vi "RotateView.vi"(8 "error in (no error)":errorcluster, 9 "Pitch":sgl, 10 "Yaw":sgl, 11 "3D Scene in":refnum<class "3D Scene.lvclass">) -> (0 "error out":errorcluster, 3 "3D Scene out":refnum<class "3D Scene.lvclass">)   [LabVIEW 2015, in "3D Scene.lvclass"]
uses:
  3D Scene.lvclass
  3D Scene.lvclass/3D Scene.ctl
  <vilib>/Analysis/baseanly.llb/Real A x B.vi
  <vilib>/Analysis/baseanly.llb/Vector x A.vi
  <vilib>/Analysis/NI_AALBase.lvlib
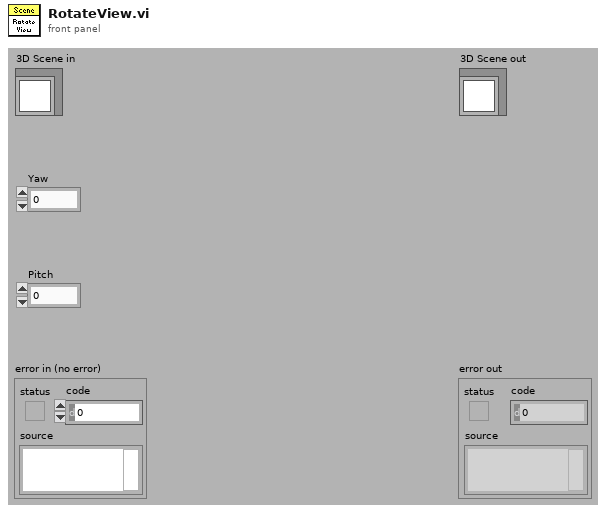
[diagram p1: front panel]
types:
  T1 = typedef "NI_Matrix.lvlib/RealMatrix.ctl" = dbl[][]
  T2 = typedef "3D Point.ctl" = cluster{"X":sgl, "Y":sgl, "Z":sgl}
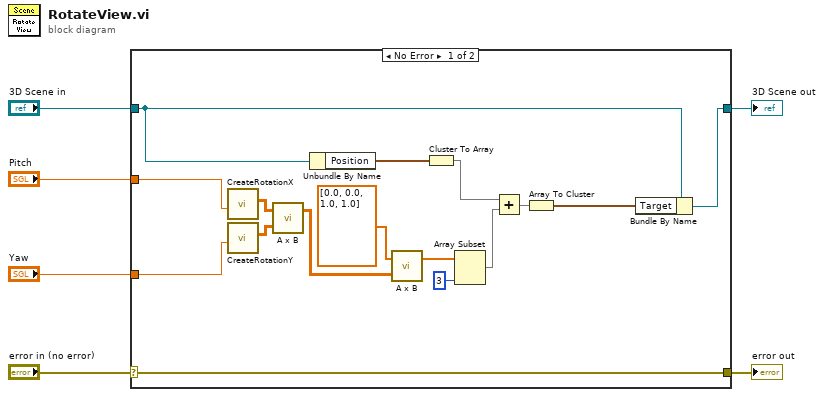
[diagram p0: block diagram]
diagram:
  n1 = case shown="No Error" "error in (no error)" {
    selector: "error in (no error)" -> [w22 w24]
    tunnel: [w22 w24] -> w5
    tunnel: [w16 w23] -> w3
    tunnel: "3D Scene in" -> [w17 w23]
    tunnel: "Pitch" -> [w19 _]
    tunnel: "Yaw" -> [w18 _]
    frame No Error {
      n2 = call "CreateRotationX.vi"("radians"=w19) -> ("modelview rotated"=w10:T1)  [unwired: 8 in, 2 out]
      n3 = call "CreateRotationY.vi"("radians"=w18) -> ("modelview rotated"=w9:T1)  [unwired: 8 in, 2 out]
      n4 = call-poly <vilib>:"A x B.vi"("B"=w9, "A"=w10) -> ("A x B"=w7:T1)  [unwired: 1 out]
      n5 = Unbundle By Name(w17) -> ("Position"=w20:T2)
      n6 = call-poly <vilib>:"A x B.vi"("Matrix A"=w7, "Vector V'"=dbl[] [0.0, 0.0, 1.0, 1.0]) -> ("V' x A"=w14:dbl[])  [unwired: 1 out]
      n7 = Cluster To Array(cluster=w20) -> (array=w12:sgl[])
      n8 = Array Subset(array=w14, length=3) -> (w13:dbl[])  [unwired: 1 in]
      n9 = Add(x=w12, y=w13) -> (x+y=w11:dbl[])
      n10 = Array To Cluster(array=w11) -> (cluster=w15:cluster{"[0]":dbl, "[1]":dbl, "[2]":dbl})
      n11 = Bundle By Name(cluster=w17, "Target"=w15) -> (w16:refnum<class "3D Scene.lvclass">)
    }
    frame Error {
    }
  }
  "error out" <- w5
  "3D Scene out" <- w3
